vi "Initialize.vi"(8 "error in (no error)":errorcluster, 10 "Angle-Value Pairs":T1[](array[typedef]), 11 "LinearInterpolation in":refnum<class "LinearInterpolation.lvclass">) -> (0 "error out":errorcluster, 3 "LinearInterpolation out":refnum<class "LinearInterpolation.lvclass">)   [LabVIEW 2013, in "LinearInterpolation.lvclass"]
uses:
  LinearInterpolation.lvclass
  AngleValuePair.ctl
  LinearInterpolation.lvclass/LinearInterpolation.ctl
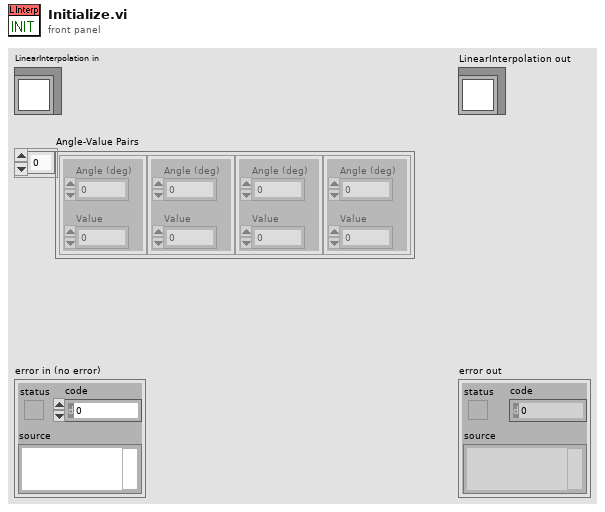
[diagram p1: front panel]
types:
  T1 = typedef "AngleValuePair.ctl" = cluster{"Angle (deg)":dbl, "Value":dbl}
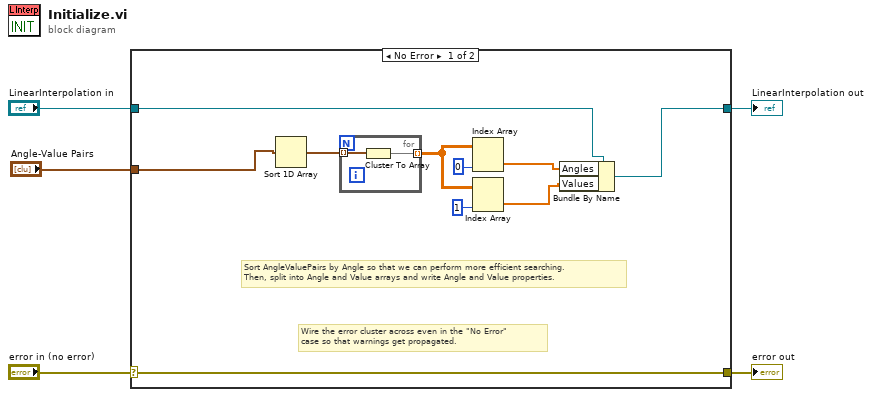
[diagram p0: block diagram]
diagram:
  n1 = case shown="No Error" "error in (no error)" {
    selector: "error in (no error)" -> [w15 w19]
    tunnel: [w15 w19] -> w4
    tunnel: [w9 w18] -> w2
    tunnel: "LinearInterpolation in" -> [w10 w18]
    tunnel: "Angle-Value Pairs" -> [w8 _]
    frame No Error {
      # "Sort AngleValuePairs by Angle so that we can perform more efficient searching.\nThen, split into Angle and Value arrays and write Angle and Value properties."
      # "Wire the error cluster across even in the \"No Error\"\ncase so that warnings get propagated."
      n2 = Sort 1D Array(array=w8) -> (sorted array=w14:T1[])
      n3 = for {
        tunnel: w14 -> [w16] mode=indexing
        tunnel: [w17] -> w11 mode=indexing
        n4 = Cluster To Array(cluster=w16) -> (array=w17:dbl[])
      }
      n5 = Index Array(array=w11, index (col)=0) -> (element=w7:dbl[])  [unwired: 1 in]
      n6 = Index Array(array=w11, index (col)=1) -> (element=w6:dbl[])  [unwired: 1 in]
      n7 = Bundle By Name(cluster=w10, "Angles"=w7, "Values"=w6) -> (w9:refnum<class "LinearInterpolation.lvclass">)
    }
    frame Error {
    }
  }
  "error out" <- w4
  "LinearInterpolation out" <- w2
